vi "Get ID.vi"(8 "error in (no error)":errorcluster, 11 "Expense Summary in":refnum<class "Expense Summary.lvclass">) -> (0 "error out":errorcluster, 2 "goal_id":i32, 3 "Expense Summary out":refnum<class "Expense Summary.lvclass">)   [LabVIEW 2018, in "Expense Summary.lvclass"]
uses:
  Expense Summary.lvclass
  Expense Summary.lvclass/Expense Summary.ctl
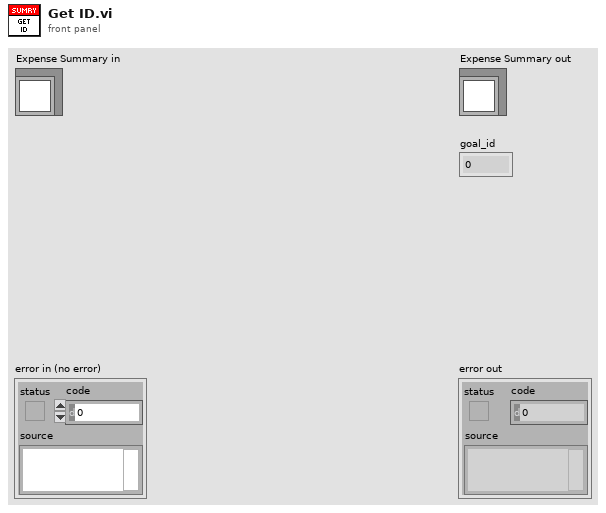
[diagram p1: front panel]
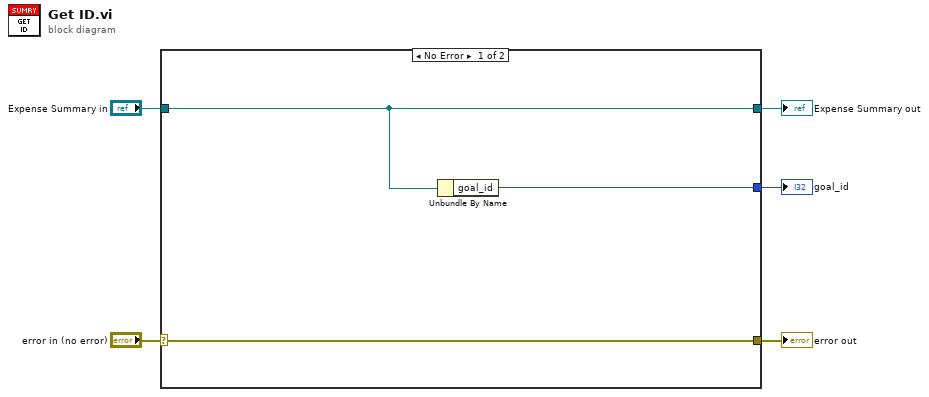
[diagram p0: block diagram]
diagram:
  n1 = case shown="No Error" "error in (no error)" {
    selector: "error in (no error)" -> [w8 w10]
    tunnel: [w8 w10] -> w4
    tunnel: [w7 w9] -> w2
    tunnel: "Expense Summary in" -> [w7 w9]
    tunnel: [w6 _] -> w1
    frame No Error {
      n2 = Unbundle By Name(w7) -> ("goal_id"=w6:i32)
    }
    frame Error {
    }
  }
  "error out" <- w4
  "Expense Summary out" <- w2
  "goal_id" <- w1
